vi "CostSavings.vi"() -> ()   [LabVIEW 2016]
panel:
  out "Savings":dbl
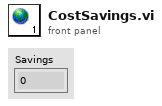
[diagram p1: front panel]
diagram:
